vi "写自动测试编号.vi"(8 "共多少路":i32, 10 "测试事项":string, 11 "编号":i32) -> (2 "输出字符串":string)   [LabVIEW 2010]
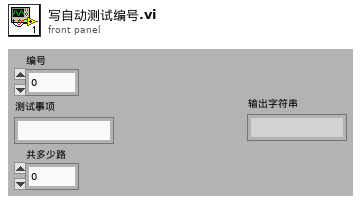
[diagram p1: front panel]
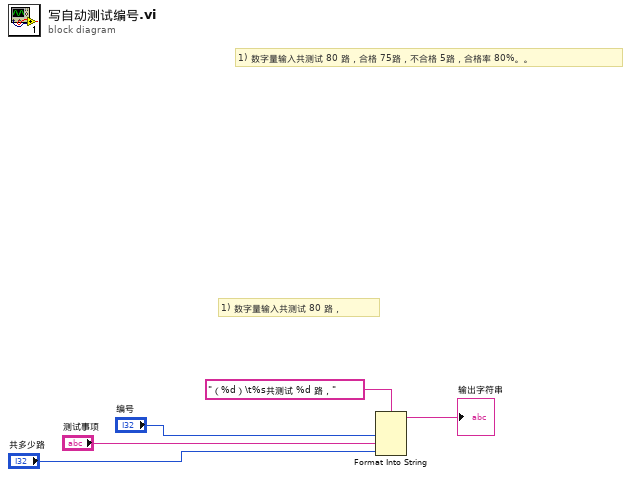
[diagram p0: block diagram]
diagram:
  # "1)\t数字量输入共测试 80 路，"
  # "1)\t数字量输入共测试 80 路，合格 75路，不合格 5路，合格率 80%。。"
  n1 = Format Into String(format string="（%d）\t%s共测试 %d 路，", "编号", "测试事项", "共多少路") -> (resulting string=→"输出字符串":string)  [unwired: 2 in, 1 out]
